vi "Complete Multipart Upload.vi"(4 "Region":T1, 8 "error in (no error)":errorcluster, 11 "Multipart Upload RefNum in":T3) -> (0 "error out":errorcluster, 1 "Version ID":string, 2 "CompleteMultipartUploadResult":T2, 3 "Multipart Upload RefNum out":T3)   [LabVIEW 2015, in "LV Interface for Amazon S3.lvlib"]
doc: "This operation completes a multipart upload by assembling previously uploaded parts. <B>You must initiate a multipart upload</B> (see Initiate Multipart Upload.vi) <B> and upload all parts before you complete a multipart upload</B>. <B>After</B> that, you have to <B>free up resources</B> on your system <B>by closing the multipart upload reference</B> (see Close Multipart Upload Reference.vi)"
uses:
  LV Interface for Amazon S3.lvlib
  Typedefs/AMZ_S3_Multipart Upload RefNum.ctl
  Typedefs/AMZ_S3_Multipart Upload RefNum Enum.ctl
  Typedefs/AMZ_S3_API_CompleteMultipartUploadResult.ctl
  Typedefs/AMZ_S3_LocationConstraint.ctl
  Typedefs/AMZ_S3_HTTP Header-Value pair.ctl
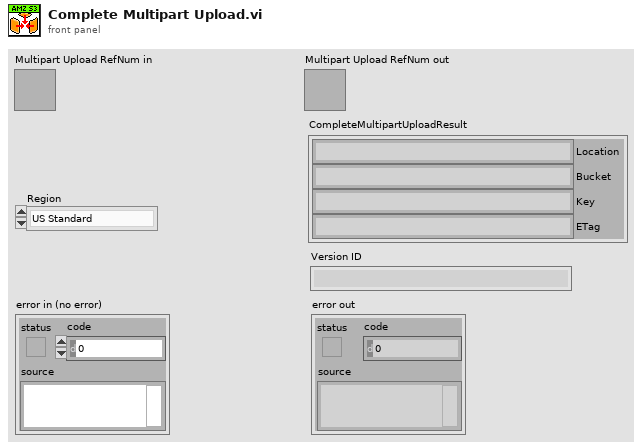
[diagram p1: front panel]
types:
  T1 = typedef "LV Interface for Amazon S3.lvlib/AMZ_S3_LocationConstraint.ctl" = enum16{"US Standard", "us-east-2", "us-west-1", "us-west-2", "ap-northeast-1", "ap-northeast-2", "ap-southeast-1", "ap-southeast-2", "ca-central-1", "eu-central-1", "eu-west-1", "eu-west-2", "sa-east-1"}
  T2 = typedef "LV Interface for Amazon S3.lvlib/AMZ_S3_API_CompleteMultipartUploadResult.ctl" = cluster{"Location":string, "Bucket":string, "Key":string, "ETag":string}
  T3 = typedef "LV Interface for Amazon S3.lvlib/AMZ_S3_Multipart Upload RefNum.ctl" = refnum<k1>
  T4 = typedef "LV Interface for Amazon S3.lvlib/AMZ_S3_HTTP Header-Value pair.ctl" = cluster{"Header":string, "Value":string}
  T5 = typedef "LV Interface for Amazon S3.lvlib/AMZ_S3_Multipart Upload Data.ctl" = cluster{"Object":string, "Bucket":string, "UploadID":string, "Parts":T6[]}
  T6 = typedef "LV Interface for Amazon S3.lvlib/AMZ_S3_Multipart Upload Part Data.ctl" = cluster{"PartNumber":u16, "Lat modified":timestamp, "ETag":string, "Size":u64}
  T7 = cluster{"format string":string, "UploadID":string}
  T8 = cluster{"format string":string, "UploadID":string}[]
  T9 = typedef "LV Interface for Amazon S3.lvlib/AMZ_S3_Call Results.ctl" = enum16{"Success", "UndefinedError", "AccessDenied", "AccountProblem", "AmbiguousGrantByEmailAddress", "BadDigest", "BucketAlreadyExists", "BucketAlreadyOwnedByYou", "BucketNotEmpty", "CredentialsNotSupported", "CrossLocationLoggingProhibited", "EntityTooSmall", "EntityTooLarge", "ExpiredToken", "IllegalVersioningConfigurationException", "IncompleteBody", "IncorrectNumberOfFilesInPostRequest", "InlineDataTooLarge", "InternalError", "InvalidAccessKeyId", "InvalidAddressingHeader", "InvalidArgument", "InvalidBucketName", "InvalidDigest", "InvalidLocationConstraint", "InvalidPart", "InvalidPartOrder", "InvalidPayer", "InvalidPolicyDocument", "InvalidRange", "InvalidSecurity", "InvalidSOAPRequest", "InvalidStorageClass", "InvalidTargetBucketForLogging", "InvalidToken", "InvalidURI", "KeyTooLong", "MalformedACLError", "MalformedPOSTRequest", "MalformedXML", "MaxMessageLengthExceeded", "MaxPostPreDataLengthExceededError", "MetadataTooLarge", "MethodNotAllowed", "MissingAttachment", "MissingContentLength", "MissingRequestBodyError", "MissingSecurityElement", "MissingSecurityHeader", "NoLoggingStatusForKey", "NoSuchBucket", "NoSuchKey", "NoSuchUpload", "NoSuchVersion", "NotImplemented", "NotSignedUp", "OperationAborted", "PermanentRedirect", "PreconditionFailed", "Redirect", "RequestIsNotMultiPartContent", "RequestTimeout", "RequestTimeTooSkewed", "RequestTorrentOfBucketError", "SignatureDoesNotMatch", "SlowDown", "TemporaryRedirect", "TokenRefreshRequired", "TooManyBuckets", "UnexpectedContent", "UnresolvableGrantByEmailAddress", "UserKeyMustBeSpecified", "LabVIEWError"}
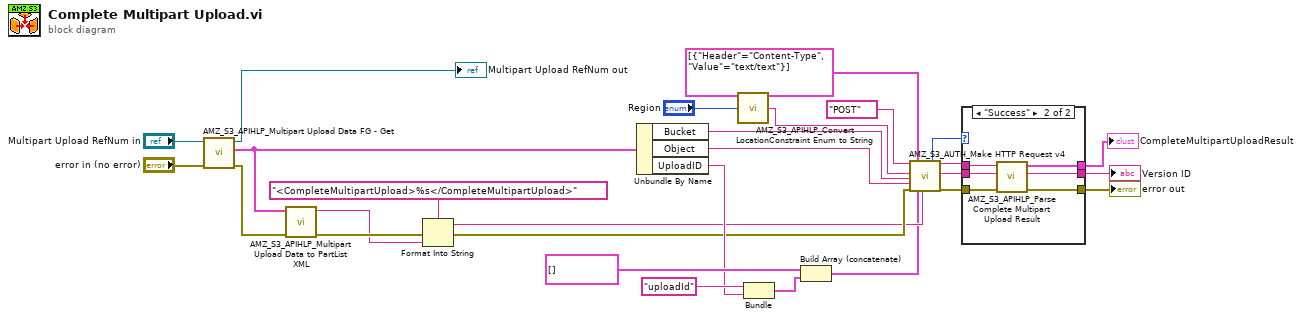
[diagram p0: block diagram]
diagram:
  n1 = call "AMZ_S3_APIHLP_Multipart Upload Data FG - Get.vi"("error in (no error)"="error in (no error)", "Multipart Upload RefNum in"="Multipart Upload RefNum in") -> ("error out"=w26:errorcluster, "Multipart Upload Data"=w25:T5, "Multipart Upload RefNum out"=→"Multipart Upload RefNum out":T3)  [unwired: 7 in]
  n2 = call "AMZ_S3_APIHLP_Multipart Upload Data to PartList XML.vi"("error in (no error)"=w26, "Multipart Upload Data"=w25) -> ("error out"=w23:errorcluster, "PartList XML"=w22:string)  [unwired: 8 in]
  n3 = Format Into String(format string="<CompleteMultipartUpload>%s</CompleteMultipartUpload>", error in=w23, w22) -> (resulting string=w5:string, error out=w6:errorcluster)  [unwired: 1 in]
  n4 = Unbundle By Name(w25) -> ("Bucket"=w8:string, "Object"=w7:string, "UploadID"=w14:string)
  n5 = call "AMZ_S3_APIHLP_Convert LocationConstraint Enum to String.vi"("Location"="Region") -> ("Location String"=w1:string)  [unwired: 4 in]
  n6 = Bundle("format string"="uploadId", "UploadID"=w14) -> (w16:T7)  [unwired: 1 in]
  n7 = Build Array (concatenate)(cluster{"item":string, "value":string}[] [] ("request parameters"), w16) -> (w4:T8)
  n8 = call "AMZ_S3_AUTH_Make HTTP Request v4.vi"("HTTP-Verb"="POST", "Region"=w1, "Bucket"=w8, "Object Key"=w7, "error in"=w6, "request headers"=T4[] [{"Header"="Content-Type", "Value"="text/text"}] ("Headers"), "request parameters"=w4, "request body"=w5) -> ("Call Result"=w10:T9, "response headers"=w11:string, "response body"=w12:string, "error out"=w13:errorcluster)  [unwired: 8 in]
  n9 = case shown="\"Success\"" w10 {
    tunnel: w13 -> [w29 w34]
    tunnel: w11 -> [_ w35]
    tunnel: w12 -> [_ w33]
    tunnel: [_ w32] -> w19
    tunnel: [w29 w31] -> w20
    tunnel: [_ w30] -> w18
    frame Default {
    }
    frame "Success" {
      n10 = call "AMZ_S3_APIHLP_Parse Complete Multipart Upload Result.vi"("error in (no error)"=w34, "Response body"=w33, "Response header"=w35) -> ("error out"=w31:errorcluster, "Version ID"=w30:string, "CompleteMultipartUploadResult"=w32:T2)  [unwired: 6 in]
    }
  }
  "error out" <- w20
  "CompleteMultipartUploadResult" <- w19
  "Version ID" <- w18
